vi "Add Game Board Component.vi"(6 "Game Board Component in":refnum<class "Game Board Component.lvclass">, 7 "Index in":i32, 11 "Game Board in":refnum<class "Game Board.lvclass">) -> (3 "Game Board out":refnum<class "Game Board.lvclass">)   [LabVIEW 2021, in "Game Board.lvclass"]
doc: "MIT Licence\nCopyright (c) 2024 David Grollier"
uses:
  Game Board.lvclass
  Game Board Component/Game Board Component.lvclass
  Game Board.lvclass/Game Board.ctl
  Game Board Component/Game Board Component.lvclass/Game Board Component.ctl
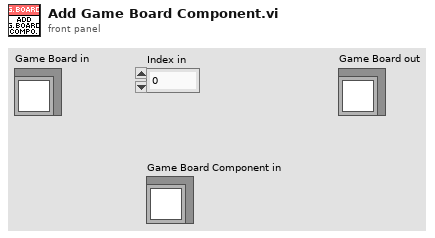
[diagram p1: front panel]
types:
  T1 = map{string, refnum<class "Game Board Component.lvclass">}
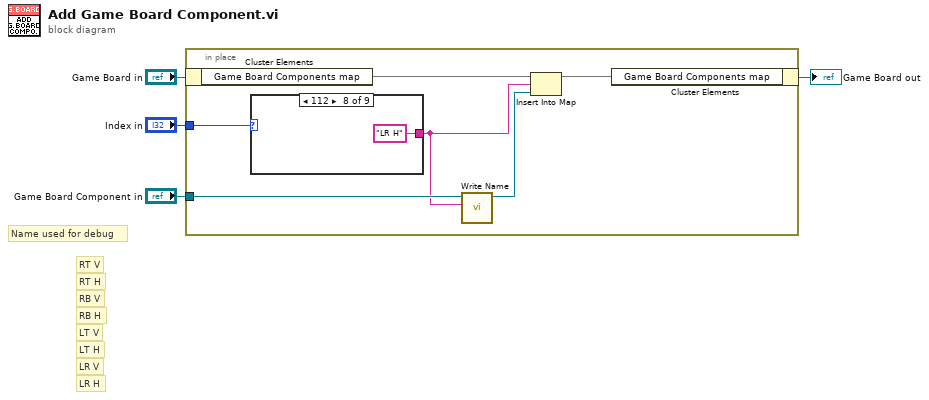
[diagram p0: block diagram]
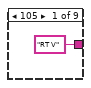
[diagram p2: hidden frame]
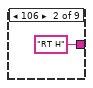
[diagram p3: hidden frame]
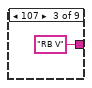
[diagram p4: hidden frame]
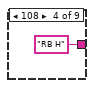
[diagram p5: hidden frame]
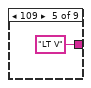
[diagram p6: hidden frame]
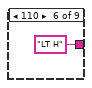
[diagram p7: hidden frame]
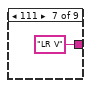
[diagram p8: hidden frame]
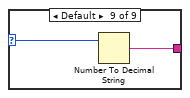
[diagram p9: hidden frame]
diagram:
  # "LR H"
  # "LR V"
  # "LT H"
  # "LT V"
  # "RB H"
  # "RB V"
  # "RT H"
  # "RT V"
  # "Name used for debug"
  n1 = in-place {
    in-place-border: "Game Board Component in" -> [w9]
    in-place-border: "Index in" -> [w7]
    n2 = in-place-cluster #1("Game Board in") -> ("Game Board Components map"=w6:T1)
    n3 = case shown="112" w7 {
      selector: w7 -> [_ _ _ _ _ _ _ _ w19]
      tunnel: ["RT V" "RT H" "RB V" "RB H" "LT V" "LT H" "LR V" "LR H" w20] -> w5
      frame 105 {
      }
      frame 106 {
      }
      frame 107 {
      }
      frame 108 {
      }
      frame 109 {
      }
      frame 110 {
      }
      frame 111 {
      }
      frame 112 {
      }
      frame Default {
        n4 = Number To Decimal String(number=w19) -> (decimal integer string=w20:string)  [unwired: 1 in]
      }
    }
    n5 = call "Write Name.vi"("Name"=w5, "Game Board Component in"=w9) -> ("Game Board Component out"=w8:refnum<class "Game Board Component.lvclass">)  [unwired: 9 in]
    n6 = Insert Into Map(map in=w6, key=w5, value=w8) -> (map out=w10:T1)  [unwired: 2 out]
    n7 = in-place-cluster #1("Game Board Components map"=w10) -> (→"Game Board out":refnum<class "Game Board.lvclass">)
  }
